vi "DAQ 실습1_1.vi"   [LabVIEW 2020]
uses:
  <vilib>/DAQmx/configure/timing.llb/DAQmx Timing (Sample Clock).vi
  <vilib>/DAQmx/create/channels.llb/DAQmx Create Channel (AI-Voltage-Basic).vi
  <vilib>/DAQmx/read.llb/DAQmx Read (Analog 1D DBL 1Chan NSamp).vi
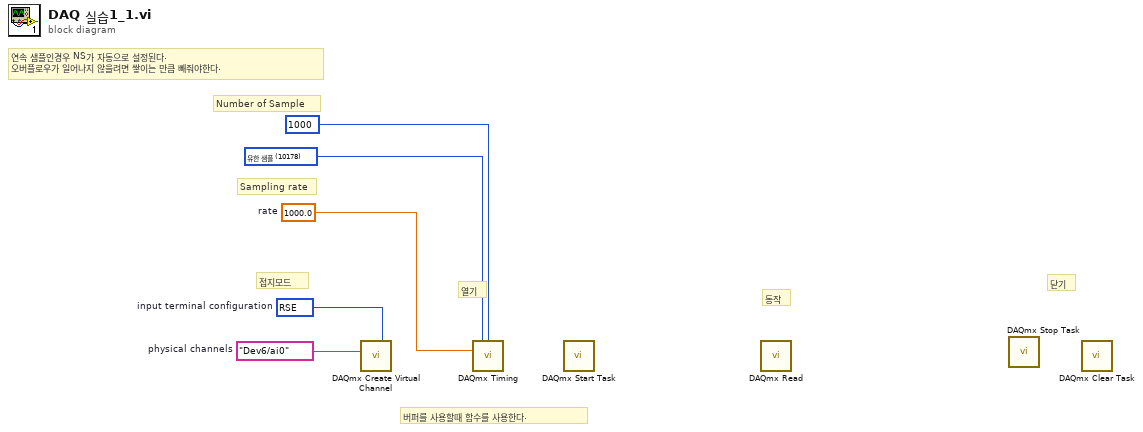
[diagram p0: block diagram]
diagram:
  w2 = 10178 items=["유한 샘플"=10178, "연속 샘플"=10123, "하드웨어 타이밍에 의한 단일 포인트"=12522] ("sample mode")
  w3 = 1000.0  # rate
  w4 = 10083 items=["기본"=-1, "RSE"=10083, "NRSE"=10078, "차동"=10106, "유사 차동"=12529]  # input terminal configuration
  w5 = tag "Dev6/ai0"  # physical channels
  # "연속 샘플인경우 NS가 자동으로 설정된다.\n오버플로우가 일어나지 않을려면 쌓이는 만큼 빼줘야한다."
  # "Number of Sample"
  # "Sampling rate"
  # "버퍼를 사용할때 함수를 사용한다."
  # "접지모드"
  # "닫기"
  # "동작"
  # "열기"
  n1 = call-poly <vilib>:"DAQmx Create Virtual Channel.vi"("input terminal configuration"=w4, "physical channels"=w5) -> ()  [unwired: 12 in, 2 out]
  n2 = call-poly <vilib>:"DAQmx Timing.vi"("sample mode"=w2, "samples per channel"=1000, "rate"=w3) -> ()  [unwired: 11 in, 2 out]
  n3 = call <vilib>:"DAQmx Start Task.vi"() -> ()  [unwired: 14 in, 2 out]
  n4 = call-poly <vilib>:"DAQmx Read.vi"() -> ()  [unwired: 13 in, 3 out]
  n5 = call <vilib>:"DAQmx Stop Task.vi"() -> ()  [unwired: 14 in, 2 out]
  n6 = call <vilib>:"DAQmx Clear Task.vi"() -> ()  [unwired: 15 in, 1 out]
